vi "Turn.vi"(8 "error in":errorcluster) -> (0 "error out":errorcluster, 3 "turn":dbl)   [LabVIEW 2014]
uses:
  Global Objects.vi
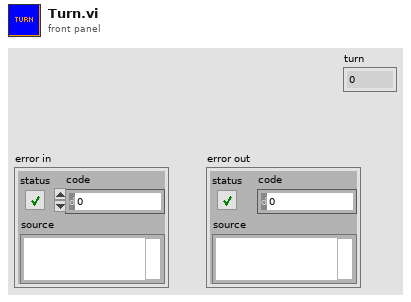
[diagram p1: front panel]
types:
  T1 = typedef "Teleop Commands.ctl" = cluster{"Throttle":dbl, "Turn":dbl, "Up Shift Commanded":bool, "Down Shift Commanded":bool}
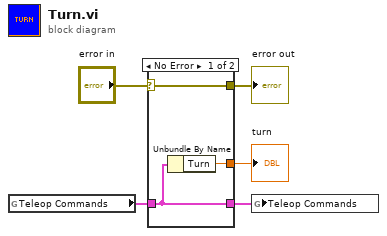
[diagram p0: block diagram]
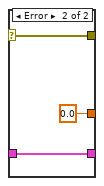
[diagram p2: hidden frame]
diagram:
  n1 = global read "Global Objects.vi" "Teleop Commands"() -> (w3:T1)
  n2 = case shown="No Error" "error in" {
    selector: "error in" -> [w8 w11]
    tunnel: [w8 w11] -> w4
    tunnel: [w7 w10] -> w2
    tunnel: w3 -> [w7 w10]
    tunnel: [w6 0.0 ("joyout")] -> w1
    frame No Error {
      n3 = Unbundle By Name(w7) -> ("Turn"=w6:dbl)
    }
    frame Error {
    }
  }
  "error out" <- w4
  "turn" <- w1
  n4 = global write "Global Objects.vi" "Teleop Commands"(w2) -> ()
